vi "Service Mode Entry.vi"(0 "GEA2 Reference In":refnum<k24>, 5 "Model":enum16{"HE", "LE"}(ring)=enum."LE", 11 "Error In":errorcluster) -> (4 "GEA2 Reference Out":refnum<k24>, 6 "Pass/Fail?":bool, 8 "Report Text":string, 15 "Error Out":errorcluster)   [LabVIEW 2016, in "Centauro.lvlib"]
doc: "Use this VI to enter service mode."
uses:
  Projects/Centauro.lvlib
  Q:/Common/DLLs/GEA3/GeaCommunication.dll
  Common/DLLs/GEA3/GeaCommunication.dll
  Common/LabVIEW GEA2 Toolkit/LabVIEW_GEA2_Toolkit.lvlibp/type defs/Source_Destination.ctl
  Common/LabVIEW GEA2 Toolkit/LabVIEW_GEA2_Toolkit.lvlibp/type defs/ERD Read Data In.ctl
  Common/LabVIEW GEA2 Toolkit/LabVIEW_GEA2_Toolkit.lvlibp/type defs/Data Type.ctl
  Common/LabVIEW GEA2 Toolkit/LabVIEW_GEA2_Toolkit.lvlibp/type defs/ERD Write Data In.ctl
  type defs/Encoder Position.ctl
  Tools/Laundry/Centauro Tool/Centauro Tool Support/type defs/Event Sequence.ctl
  type defs/Service Mode Pointer.ctl
  Common/LabVIEW GEA2 Toolkit/LabVIEW_GEA2_Toolkit.lvlibp
panel:
  in  "Standalone?":bool
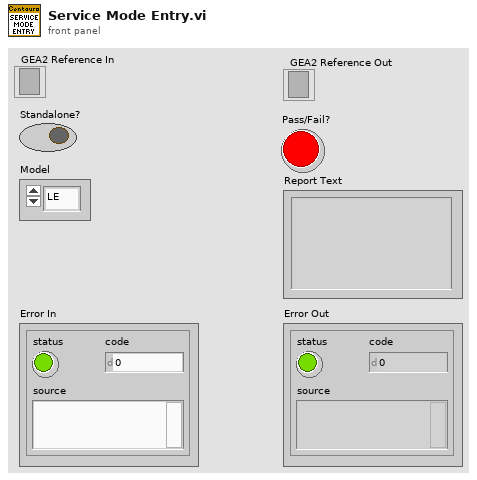
[diagram p1: front panel]
types:
  T1 = typedef "LabVIEW_GEA2_Toolkit.lvlibp/ERD Write Data In.ctl" = cluster{"ERD Number":u16, "Data Type":T2, "Data":string}
  T2 = typedef "LabVIEW_GEA2_Toolkit.lvlibp/Data Type.ctl" = enum16{"string", "boolean", "uint8_t", "uint16_t", "uint32_t", "uint64_t", "int8_t", "int16_t", "int32_t", "int64_t"}
  T3 = typedef "LabVIEW_GEA2_Toolkit.lvlibp/ERD Read Data In.ctl" = cluster{"ERD Number":u16, "Data Type":T2}
  T4 = typedef "LabVIEW_GEA2_Toolkit.lvlibp/Source_Destination.ctl" = cluster{"Source":u8, "Destination":u8}
  T5 = typedef "Service Mode Pointer.ctl" = enum16{"Set ", "Get"}
  T6 = typedef "Event Sequence.ctl" = enum16{"Nothing", "StartButtonPress", "StartButtonRelease", "DeepRinseKeyPress", "DeepRinseKeyRelease", "CycleKnobPosition0", "CycleKnobPosition1", "CycleKnobPosition2", "CycleKnobPosition3", "CycleKnobPosition4", "CycleKnobPosition5", "CycleKnobPosition6", "CycleKnobPosition7", "CycleKnobPosition8", "CycleKnobPosition9", "CycleKnobPosition10", "CycleKnobPosition11", "OptionKnob1Position0", "OptionKnob1Position1", "OptionKnob1Position2", "OptionKnob1Position3", "OptionKnob1Position4", "OptionKnob1Position5", "OptionKnob2Position0", "OptionKnob2Position1", "OptionKnob2Position2", "OptionKnob2Position3", "OptionKnob2Position4"}
  T7 = typedef "Centauro.lvlib/Encoder Position.ctl" = enum16{"Position 0", "Position 1", "Position 2", "Position 3", "Position 4", "Position 5", "Position 6", "Position 7", "Position 8", "Position 9", "Position 10", "Position 11", "Position 12", "Position 13", "Clear / Reset"}
  T8 = enum16{"CycleKnobPosition0", "CycleKnobPosition1", "CycleKnobPosition2", "CycleKnobPosition3", "CycleKnobPosition4", "CycleKnobPosition5", "CycleKnobPosition6", "CycleKnobPosition7", "CycleKnobPosition8", "CycleKnobPosition9", "CycleKnobPosition10", "CycleKnobPosition11"}[]
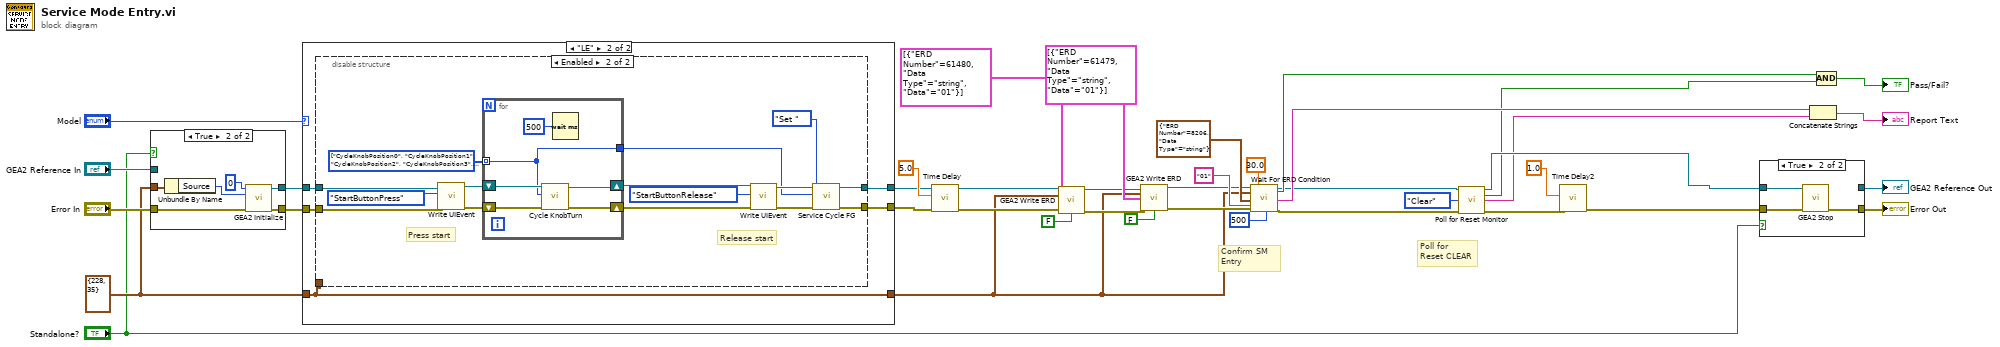
[diagram p0: block diagram]
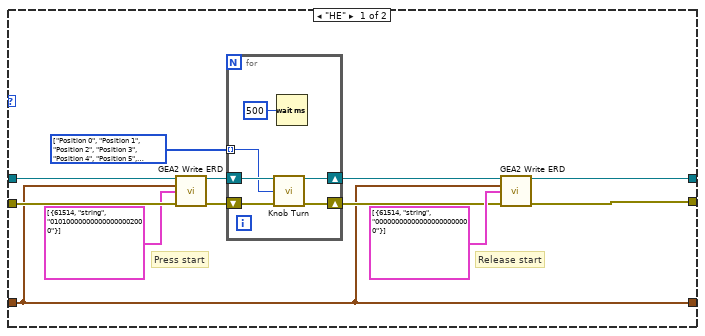
[diagram p2: hidden frame]
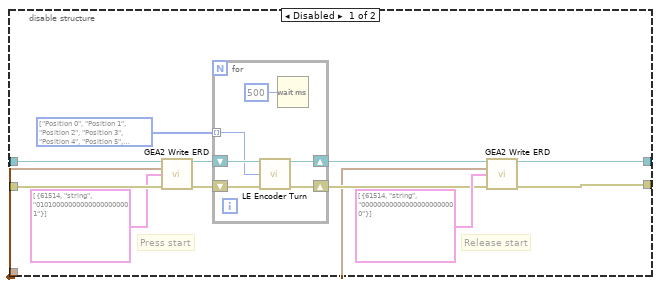
[diagram p3: hidden frame]
diagram:
  w33 = T4 {"Source"=228, "Destination"=35} ("GEA Inputs")
  # "Confirm SM \nEntry"
  # "Poll for\nReset CLEAR"
  n1 = case shown="True" "Standalone?" {
    tunnel: "Error In" -> [w40 w47]
    tunnel: [w40 w46] -> w35
    tunnel: "GEA2 Reference In" -> [w41 _]
    tunnel: [w41 w45] -> w36
    tunnel: w33 -> [_ w43]
    frame False {
    }
    frame True {
      n2 = Unbundle By Name(w43) -> ("Source"=w44:u8)
      n3 = call "GEA2 Initialize.vi"("Board Index"=0, "Source Address"=w44, "error in"=w47) -> ("GEA2 Reference Out"=w45:refnum<k24>, "error out"=w46:errorcluster)  [unwired: 10 in, 1 out]
    }
  }
  n4 = case shown="\"LE\"" "Model" {
    tunnel: w36 -> [w56 w70]
    tunnel: w35 -> [w55 w69]
    tunnel: w33 -> [w48 w66]
    tunnel: [w50 w68] -> w15
    tunnel: [w49 w67] -> w32
    tunnel: [w48 w66] -> w1
    frame "HE" {
      w59 = T7[] [enum."Position 0", enum."Position 1", enum."Position 2", enum."Position 3", enum."Position 4", enum."Position 5", enum."Position 6", enum."Position 7"] items=["Position 0", "Position 1", "Position 2", "Position 3", "Position 4", "Position 5", "Position 6", "Position 7", "Position 8", "Position 9", "Position 10", "Position 11", "Position 12", "Position 13", "Clear / Reset"]
      # "Release start"
      # "Press start"
      n5 = call "GEA2 Write ERD.vi"("GEA2 Reference In"=w56, "GEA Inputs"=w48, "Write ERD List"=T1[] [{"ERD Number"=61514, "Data Type"=enum."string", "Data"="010100000000000000002000"}], "Error In"=w55) -> ("GEA2 Reference Out"=w58:refnum<k24>, "Error Out"=w57:errorcluster)  [unwired: 9 in, 1 out]
      n6 = for {
        shift-right: [w64] -> w51
        shift-left: w58 -> [w65]
        shift-right: [w62] -> w52
        shift-left: w57 -> [w63]
        tunnel: w59 -> [w61] mode=indexing
        n7 = call "Knob Turn.vi"("GEA2 Reference In"=w65, "Button"=w61, "Error In"=w63) -> ("GEA2 Reference Out"=w64:refnum<k24>, "Error Out"=w62:errorcluster)  [unwired: 11 in]
        n8 = Wait (ms)(milliseconds to wait=u32 500) -> ()  [unwired: 1 out]
      }
      n9 = call "GEA2 Write ERD.vi"("GEA2 Reference In"=w51, "GEA Inputs"=w48, "Write ERD List"=T1[] [{"ERD Number"=61514, "Data Type"=enum."string", "Data"="000000000000000000000000"}], "Error In"=w52) -> ("GEA2 Reference Out"=w50:refnum<k24>, "Error Out"=w49:errorcluster)  [unwired: 9 in, 1 out]
    }
    frame "LE" {
      n10 = disable-structure shown="Enabled" {
        disable-tunnel: w70 -> [w79 w95]
        disable-tunnel: w69 -> [w78 w94]
        disable-tunnel: [w73 w96] -> w68
        disable-tunnel: [w72 w92] -> w67
        disable-tunnel: w66 -> [w71 _]
        frame Disabled {
          w82 = T7[] [enum."Position 0", enum."Position 1", enum."Position 2", enum."Position 3", enum."Position 4", enum."Position 5", enum."Position 6"] items=["Position 0", "Position 1", "Position 2", "Position 3", "Position 4", "Position 5", "Position 6", "Position 7", "Position 8", "Position 9", "Position 10", "Position 11", "Position 12", "Position 13", "Clear / Reset"]
          # "Release start"
          # "Press start"
          n11 = call "GEA2 Write ERD.vi"("GEA2 Reference In"=w79, "GEA Inputs"=w71, "Write ERD List"=T1[] [{"ERD Number"=61514, "Data Type"=enum."string", "Data"="010100000000000000000001"}], "Error In"=w78) -> ("GEA2 Reference Out"=w81:refnum<k24>, "Error Out"=w80:errorcluster)  [unwired: 9 in, 1 out]
          n12 = for {
            shift-right: [w87] -> w74
            shift-left: w81 -> [w88]
            shift-right: [w85] -> w75
            shift-left: w80 -> [w86]
            tunnel: w82 -> [w84] mode=indexing
            n13 = call "LE Encoder Turn.vi"("GEA2 Reference In"=w88, "Button"=w84, "Error In"=w86) -> ("GEA2 Reference Out"=w87:refnum<k24>, "Error Out"=w85:errorcluster)  [unwired: 11 in]
            n14 = Wait (ms)(milliseconds to wait=u32 500) -> ()  [unwired: 1 out]
          }
          n15 = call "GEA2 Write ERD.vi"("GEA2 Reference In"=w74, "GEA Inputs"=w71, "Write ERD List"=T1[] [{"ERD Number"=61514, "Data Type"=enum."string", "Data"="000000000000000000000000"}], "Error In"=w75) -> ("GEA2 Reference Out"=w73:refnum<k24>, "Error Out"=w72:errorcluster)  [unwired: 9 in, 1 out]
        }
        frame Enabled {
          w89 = T8 [enum."CycleKnobPosition0", enum."CycleKnobPosition1", enum."CycleKnobPosition2", enum."CycleKnobPosition3", enum."CycleKnobPosition4", enum."CycleKnobPosition5", enum."CycleKnobPosition6"] items=["CycleKnobPosition0", "CycleKnobPosition1", "CycleKnobPosition2", "CycleKnobPosition3", "CycleKnobPosition4", "CycleKnobPosition5", "CycleKnobPosition6", "CycleKnobPosition7", "CycleKnobPosition8", "CycleKnobPosition9", "CycleKnobPosition10", "CycleKnobPosition11"] ("Array")
          # "Release start"
          # "Press start"
          n16 = call "Write UIEvent.vi"("Error In"=w94, "Event ID"=Event_Sequence."StartButtonPress", "GEA2 Reference In"=w95) -> ("Error Out"=w102:errorcluster, "GEA2 Reference Out"=w101:refnum<k24>)  [unwired: 7 in]
          n17 = for {
            shift-right: [w106] -> w99
            shift-left: w101 -> [w107]
            shift-right: [w104] -> w98
            shift-left: w102 -> [w105]
            tunnel: w89 -> [w103] mode=indexing
            tunnel: [w103] -> w91
            n18 = call "Cycle KnobTurn.vi"("Error In"=w105, "Cycle Knob"=w103, "GEA2 Reference In"=w107) -> ("Error Out"=w104:errorcluster, "GEA2 Reference Out"=w106:refnum<k24>)  [unwired: 7 in]
            n19 = Wait (ms)(milliseconds to wait=u32 500) -> ()  [unwired: 1 out]
          }
          n20 = call "Write UIEvent.vi"("Error In"=w98, "Event ID"=Event_Sequence."StartButtonRelease", "GEA2 Reference In"=w99) -> ("Error Out"=w93:errorcluster, "GEA2 Reference Out"=w96:refnum<k24>)  [unwired: 7 in]
          n21 = call "Service Cycle FG.vi"("Error In"=w93, "Cycle Knob"=w91, "Action"=Service_Mode_Pointer."Set ") -> ("Error Out"=w92:errorcluster)  [unwired: 7 in, 1 out]
        }
      }
    }
  }
  n22 = call "Time Delay"("error in (no error)"=w32, "Delay Time (s)"=5.0) -> ("error out"=w14:errorcluster)  [unwired: 9 in]
  n23 = call "GEA2 Write ERD.vi"("GEA2 Reference In"=w15, "GEA Inputs"=w1, "Write ERD List"=T1[] [{"ERD Number"=61480, "Data Type"=enum."string", "Data"="01"}], "Error In"=w14, "Verify ERD Response?"=FALSE) -> ("GEA2 Reference Out"=w11:refnum<k24>, "Error Out"=w9:errorcluster)  [unwired: 8 in, 1 out]
  n24 = call "GEA2 Write ERD.vi"("GEA2 Reference In"=w11, "GEA Inputs"=w1, "Write ERD List"=T1[] [{"ERD Number"=61479, "Data Type"=enum."string", "Data"="01"}], "Error In"=w9, "Verify ERD Response?"=FALSE) -> ("GEA2 Reference Out"=w10:refnum<k24>, "Error Out"=w8:errorcluster)  [unwired: 8 in, 1 out]
  n25 = call "Wait For ERD Condition.vi"("GEA2 Reference In"=w10, "GEA Inputs"=w1, "ERD Read Data"=T3 {"ERD Number"=8206, "Data Type"=enum."string"} ("ERD Read Data In"), "Expected Low"="01", "Error In"=w8, "Timeout (s)"=30.0, "Loop Rate (ms)"=u32 500) -> ("GEA2 Reference Out"=w5:refnum<k24>, "Pass/Fail?"=w6:bool, "Report Text"=w25:string, "Error Out"=w4:errorcluster)  [unwired: 8 in, 1 out]
  n26 = call "Poll for Reset Monitor.vi"("GEA2 Reference In"=w5, "Status"=enum16{"Clear", "Set"}."Clear", "Error In"=w4) -> ("GEA2 Reference Out"=w18:refnum<k24>, "Pass/Fail?"=w3:bool, "Report Text"=w2:string, "Error Out"=w21:errorcluster)  [unwired: 8 in, 1 out]
  n27 = call "Time Delay2"("error in (no error)"=w21, "Delay Time (s)"=1.0) -> ("error out"=w19:errorcluster)  [unwired: 9 in]
  n28 = case shown="True" "Standalone?" {
    tunnel: [w110 w113] -> w39
    tunnel: w19 -> [w110 w112]
    tunnel: w18 -> [w109 w111]
    tunnel: [w109 _] -> w26
    frame False {
    }
    frame True {
      n29 = call "GEA2 Stop.vi"("GEA2 Reference In"=w111, "Error In"=w112) -> ("Error Out"=w113:errorcluster)  [unwired: 13 in]
    }
  }
  "Error Out" <- w39
  "GEA2 Reference Out" <- w26
  n30 = Concatenate Strings(w25, w2) -> (→"Report Text":string)
  n31 = Compound Arithmetic op=AND(w6, w3) -> (→"Pass/Fail?":bool)
